vi "AES DataReplay Scale Raw Data to DAC Data.vi"(8 "max voltage of AO DAC (10)":dbl=10.0, 9 "votlage at max RPM":dbl, 10 "DAC bit resolution (16)":u8=16, 11 "replay data":dbl[](array[numeric])) -> (3 "DAC data":i16[](array[numeric]))   [LabVIEW 2010, in "AES.lvlib" / "AES RT.lvlib"]
doc: "This VI takes the raw replay data and scales it to the I16 values the digital to analog converter (DAC) uses on the FPGA.\n\nNote: Set the \"Use Cycle? (F)\" input to true if your N Teeth M Missing generation loop is referencing the Cycle Angle (0-720) not the Crank Angle (0-360)"
uses:
  AES RT.lvlib
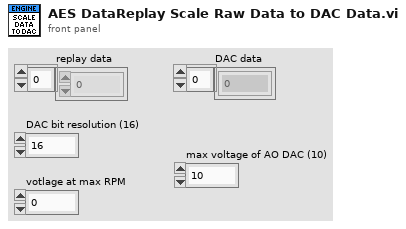
[diagram p1: front panel]
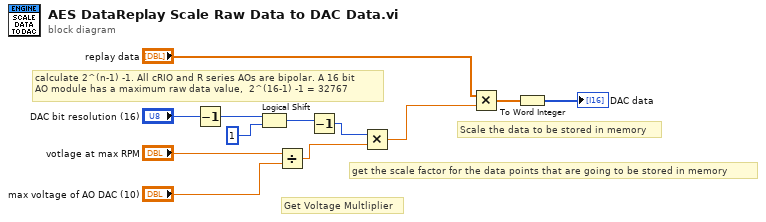
[diagram p0: block diagram]
diagram:
  # "calculate 2^(n-1) -1. All cRIO and R series AOs are bipolar. A 16 bit\nAO module has a maximum raw data value,  2^(16-1) -1 = 32767"
  # "Scale the data to be stored in memory"
  # "get the scale factor for the data points that are going to be stored in memory"
  # "Get Voltage Multliplier"
  n1 = Decrement(x="DAC bit resolution (16)") -> (x-1=w9:u8)
  n2 = Logical Shift(y=w9, x=i16 1) -> (x << y=w10:i16)
  n3 = Divide(x="votlage at max RPM", y="max voltage of AO DAC (10)") -> (x/y=w3:dbl)
  n4 = Decrement(x=w10) -> (x-1=w11:i16)
  n5 = Multiply(x=w11, y=w3) -> (x*y=w4:dbl)
  n6 = Multiply(x="replay data", y=w4) -> (x*y=w5:dbl[])
  n7 = To Word Integer(number=w5) -> (16bit integer=→"DAC data":i16[])
